vi "002 llegir de fitxer.vi"() -> ()   [LabVIEW 2019]
uses:
  <vilib>/Analysis/baseanly.llb/Mean (DBL).vi
  <vilib>/Analysis/NI_AALBase.lvlib
panel:
  out "min value":dbl
  out "max value":dbl
  out "mean":dbl format="%0.2f"
  out "Waveform Graph":dynamicdata(graph)
  in  "Search Button":bool
  in  "stop":bool
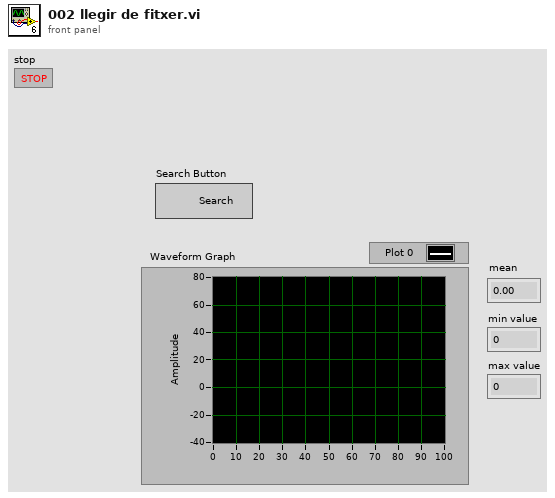
[diagram p1: front panel]
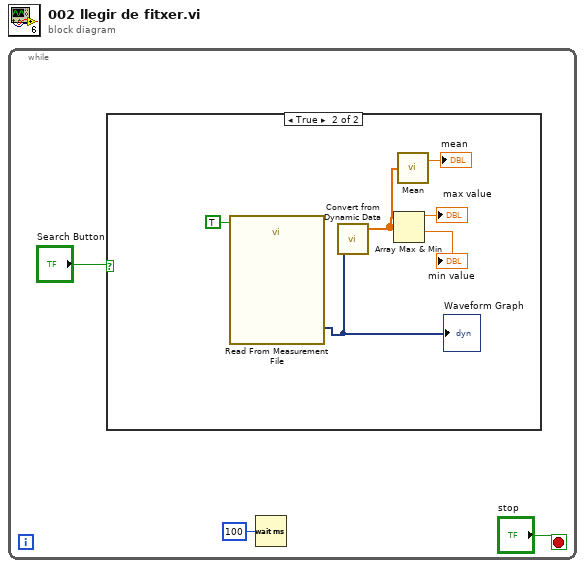
[diagram p0: block diagram]
diagram:
  n1 = while {
    stop <- "stop" stop-if-true
    n2 = case shown="True" "Search Button" {
      frame False {
      }
      frame True {
        n3 = call "Read From Measurement File"("Reset"=TRUE) -> ("Signals"=w5:dynamicdata)  [unwired: 5 in, 5 out]
        "Waveform Graph" <- w5
        n4 = call "Convert from Dynamic Data"("Dynamic Data Type"=w5) -> ("Array"=w4:dbl[])  [unwired: 3 in]
        n5 = Array Max & Min(array=w4) -> (max value=→"max value":dbl, min value=→"min value":dbl)  [unwired: 2 out]
        n6 = call-poly <vilib>:"Mean.vi"("X"=w4) -> ("mean"=→"mean":dbl)  [unwired: 1 out]
      }
    }
    n7 = Wait (ms)(milliseconds to wait=u32 100) -> ()  [unwired: 1 out]
  }
